vi "DestroyEvent.vi"(8 "error in (no error)":errorcluster, 11 "object in":refnum<class "EventMsg.lvclass">) -> (0 "error out":errorcluster, 3 "object out":refnum<class "EventMsg.lvclass">)   [LabVIEW 2014, in "EventMsg.lvclass"]
doc: "Destroy the user event reference indicated by Name."
uses:
  EventMsg.lvclass
  EventMsg.lvclass/EventMsg.ctl
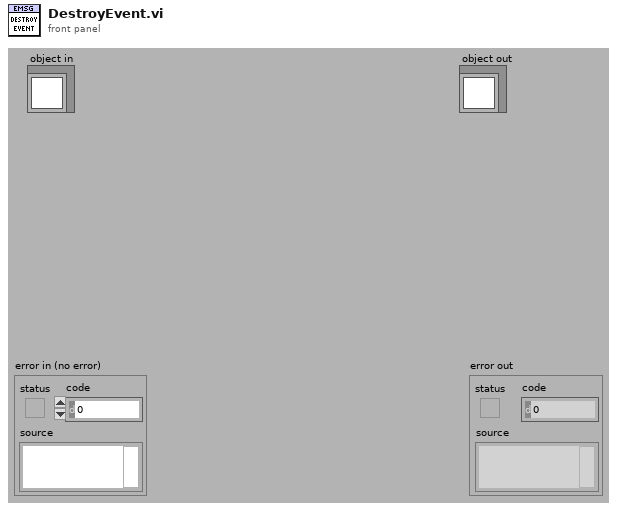
[diagram p1: front panel]
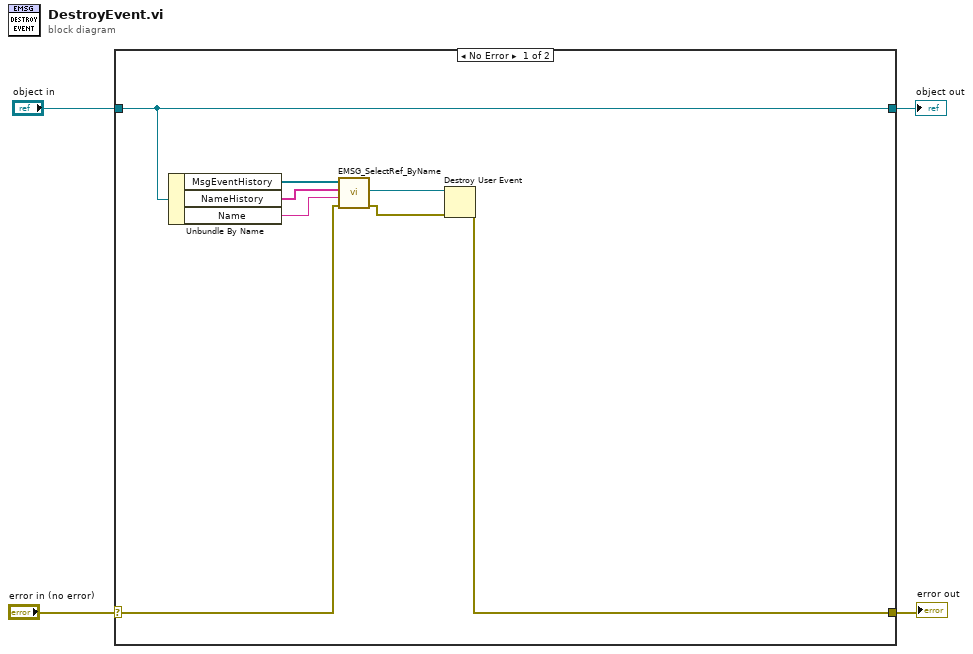
[diagram p0: block diagram]
diagram:
  n1 = case shown="No Error" "error in (no error)" {
    selector: "error in (no error)" -> [w7 w14]
    tunnel: [w11 w14] -> w3
    tunnel: [w12 w13] -> w1
    tunnel: "object in" -> [w12 w13]
    frame No Error {
      n2 = Unbundle By Name(w12) -> ("MsgEventHistory"=w9:refnum<user-event>[], "NameHistory"=w8:string[], "Name"=w5:string)
      n3 = call "EMSG_SelectRef_ByName.vi"("Error in"=w7, "Name"=w5, "NameHistory"=w8, "MsgEventHistory"=w9) -> ("Error out"=w6:errorcluster, "User Event out"=w10:refnum<user-event>)  [unwired: 6 in]
      n4 = Destroy User Event(user event=w10, error in=w6) -> (error out=w11:errorcluster)
    }
    frame Error {
    }
  }
  "error out" <- w3
  "object out" <- w1
